vi "Noyito10ChannelADC_SingleSampleAllChannels.vi"(7 "Timeout (s)":dbl=10.0, 8 "error in (no error)":errorcluster) -> (0 "error out":errorcluster, 1 "Error":bool, 2 "ADC Counts":T1, 3 "ADC Voltages":T2, 5 "Full Sample Text":string)   [LabVIEW 2020, in "NOYITO 10 Channel ADC Module Driver.lvlib"]
uses:
  NOYITO 10 Channel ADC Module Driver.lvlib
panel:
  in  "Tab Control":enum32{"Page 1", "Page 2"}(tab)
  out "readBuffer":string
  in  "STOP SAMPLING":bool
  out "#bytes at port":u32=115200
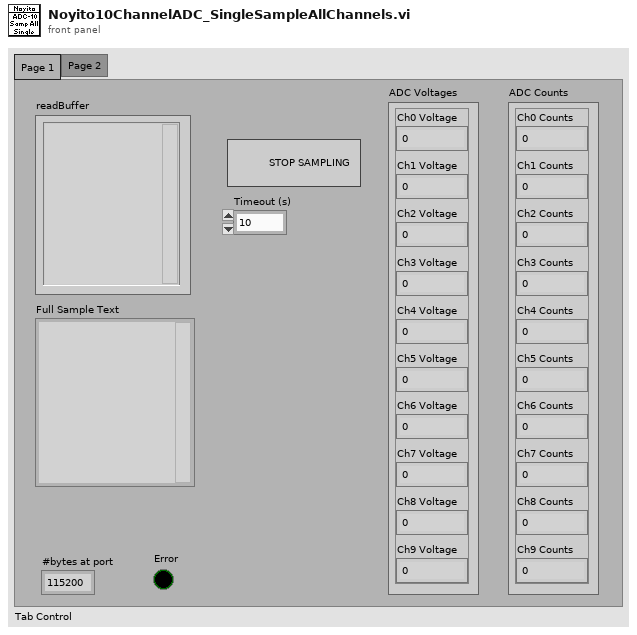
[diagram p1: front panel]
types:
  T1 = cluster{"Ch0 Counts":u16, "Ch1 Counts":u16, "Ch2 Counts":u16, "Ch3 Counts":u16, "Ch4 Counts":u16, "Ch5 Counts":u16, "Ch6 Counts":u16, "Ch7 Counts":u16, "Ch8 Counts":u16, "Ch9 Counts":u16}
  T2 = cluster{"Ch0 Voltage":dbl, "Ch1 Voltage":dbl, "Ch2 Voltage":dbl, "Ch3 Voltage":dbl, "Ch4 Voltage":dbl, "Ch5 Voltage":dbl, "Ch6 Voltage":dbl, "Ch7 Voltage":dbl, "Ch8 Voltage":dbl, "Ch9 Voltage":dbl}
  T3 = cluster{"[0]":dbl, "[1]":dbl, "[2]":dbl, "[3]":dbl, "[4]":dbl, "[5]":dbl, "[6]":dbl, "[7]":dbl, "[8]":dbl, "[9]":dbl}
  T4 = cluster{"[0]":i32, "[1]":i32, "[2]":i32, "[3]":i32, "[4]":i32, "[5]":i32, "[6]":i32, "[7]":i32, "[8]":i32, "[9]":i32}
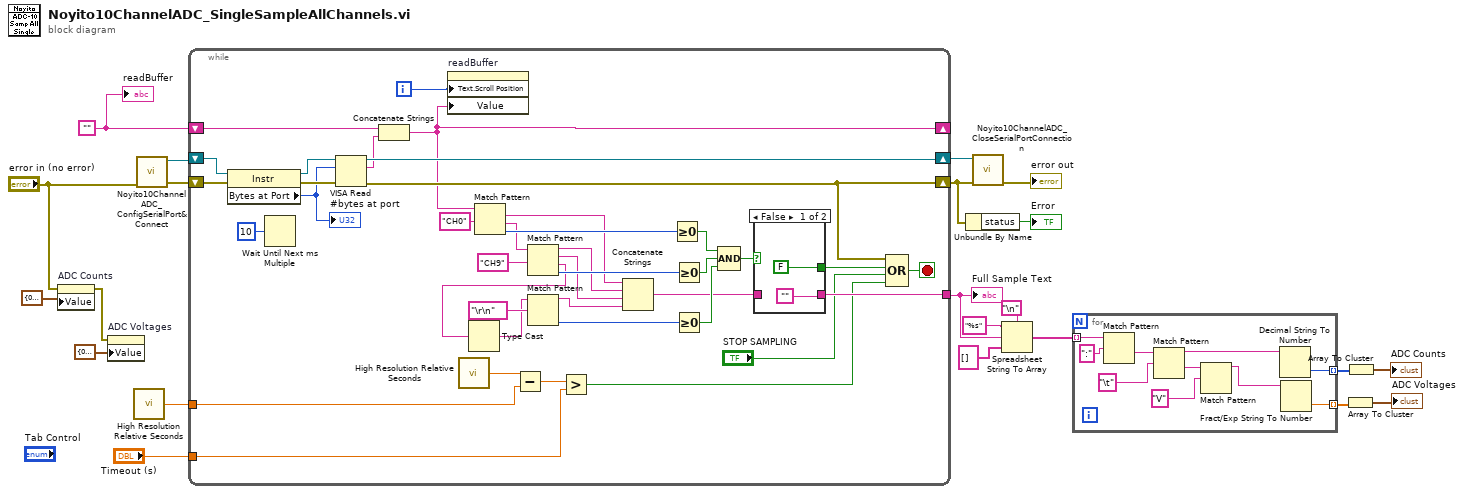
[diagram p0: block diagram]
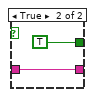
[diagram p2: hidden frame]
diagram:
  w20 = ""
  n1 = property on="ADC Counts" class="Clust (strict)"(error in="error in (no error)", "Value"=T1 {"Ch0 Counts"=0, "Ch1 Counts"=0, "Ch2 Counts"=0, "Ch3 Counts"=0, "Ch4 Counts"=0, "Ch5 Counts"=0, "Ch6 Counts"=0, "Ch7 Counts"=0, "Ch8 Counts"=0, "Ch9 Counts"=0} ("ADC Counts")) -> (error out=w1:errorcluster)  [unwired: 1 in, 1 out]
  n2 = property on="ADC Voltages" class="Clust (strict)"(error in=w1, "Value"=T2 {"Ch0 Voltage"=0.0, "Ch1 Voltage"=0.0, "Ch2 Voltage"=0.0, "Ch3 Voltage"=0.0, "Ch4 Voltage"=0.0, "Ch5 Voltage"=0.0, "Ch6 Voltage"=0.0, "Ch7 Voltage"=0.0, "Ch8 Voltage"=0.0, "Ch9 Voltage"=0.0} ("ADC Voltages")) -> ()  [unwired: 1 in, 2 out]
  n3 = call <vilib>:"High Resolution Relative Seconds.vi"() -> ("relative seconds"=w19:dbl)
  n4 = call "Noyito10ChannelADC_ConfigSerialPort&Connect.vi"("error in (no error)"="error in (no error)") -> ("error out"=w22:errorcluster, "Noyito 10Chan ADC Mod"=w21:refnum<visa-resource-name>)  [unwired: 9 in]
  n5 = while {
    shift-right: [w43] -> w6
    shift-left: w22 -> [w61]
    shift-right: [w56] -> w17
    shift-left: w21 -> [w60]
    shift-right: [w40] -> _
    shift-left: w20 -> [w53]
    tunnel: [w46] -> w16
    tunnel: w19 -> [w26]
    tunnel: "Timeout (s)" -> [w24]
    i -> [w45]
    stop <- w55 stop-if-true
    w35 = "\r\n"
    n6 = property class="Instr"(reference=w60, error in=w61) -> (reference out=w58:refnum<visa-resource-name>, error out=w59:errorcluster, "Bytes at Port"=w52:u32)
    "#bytes at port" <- w52
    n7 = Wait Until Next ms Multiple(millisecond multiple=u32 10) -> ()  [unwired: 1 out]
    n8 = VISA Read(VISA resource name=w58, byte count=w52, error in (no error)=w59) -> (VISA resource name out=w56:refnum<visa-resource-name>, read buffer=w54:string, error out=w43:errorcluster)  [unwired: 1 out]
    n9 = Concatenate Strings(w53, w54) -> (w40:string)
    n10 = property on="readBuffer" class="Str"("Text.Scroll Position"=w45, "Value"=w40) -> ()  [unwired: 2 in, 2 out]
    n11 = call <vilib>:"High Resolution Relative Seconds.vi"() -> ("relative seconds"=w27:dbl)
    n12 = Match Pattern(string=w40, regular expression="CH0") -> (match substring=w32:string, after substring=w41:string, offset past match=w51:i32)  [unwired: 1 in, 1 out]
    n13 = Subtract(x=w27, y=w26) -> (x-y=w25:dbl)
    n14 = Match Pattern(string=w41, regular expression="CH9") -> (before substring=w30:string, match substring=w29:string, after substring=w36:string, offset past match=w50:i32)  [unwired: 1 in]
    n15 = Type Cast(type=w35, x=w36) -> (*(type *) &x=w34:string)
    n16 = Match Pattern(string=w34, regular expression=w35) -> (before substring=w28:string, offset past match=w37:i32)  [unwired: 1 in, 2 out]
    n17 = Greater?(x=w25, y=w24) -> (0:w23:bool)
    n18 = Concatenate Strings(w32, w30, w29, w28) -> (w31:string)
    n19 = Greater Or Equal To 0?(x=w51) -> (x >= 0?=w48:bool)
    n20 = Greater Or Equal To 0?(x=w50) -> (x >= 0?=w49:bool)
    n21 = Greater Or Equal To 0?(x=w37) -> (x >= 0?=w33:bool)
    n22 = Compound Arithmetic op=AND(w48, w49, w33) -> (w47:bool)
    n23 = case shown="False" w47 {
      tunnel: ["" w64] -> w46
      tunnel: [FALSE TRUE] -> w44
      tunnel: w31 -> [_ w64]
      frame False {
      }
      frame True {
      }
    }
    n24 = Compound Arithmetic op=OR(w43, w44, "STOP SAMPLING", w23) -> (w55:bool)
  }
  "Full Sample Text" <- w16
  n25 = Unbundle By Name(w6) -> ("status"=→"Error":bool)
  n26 = call "Noyito10ChannelADC_CloseSerialPortConnection.vi"("error in (no error)"=w6, "Noyito 10Chan ADC Mod"=w17) -> ("error out"=→"error out":errorcluster)  [unwired: 8 in, 1 out]
  n27 = Spreadsheet String To Array(delimiter (Tab)="\n", format string="%s", spreadsheet string=w16, array type (2D Dbl)=string[] []) -> (array=w12:string[])
  n28 = for {
    tunnel: w12 -> [w75] mode=indexing
    tunnel: [w71] -> w11 mode=indexing
    tunnel: [w70] -> w10 mode=indexing
    n29 = Match Pattern(string=w75, regular expression=":") -> (after substring=w73:string)  [unwired: 1 in, 3 out]
    n30 = Match Pattern(string=w73, regular expression="\t") -> (before substring=w72:string, after substring=w69:string)  [unwired: 1 in, 2 out]
    n31 = Match Pattern(string=w69, regular expression="V") -> (before substring=w67:string)  [unwired: 1 in, 3 out]
    n32 = Decimal String To Number(string=w72) -> (number=w71:i32)  [unwired: 2 in, 1 out]
    n33 = Fract/Exp String To Number(string=w67) -> (number=w70:dbl)  [unwired: 3 in, 1 out]
  }
  n34 = Array To Cluster(array=w10) -> (cluster=→"ADC Voltages":T3)
  n35 = Array To Cluster(array=w11) -> (cluster=→"ADC Counts":T4)
  "readBuffer" <- w20
